vi "OpenDoc Browser.vi"(8 "error in (no error)":errorcluster, 10 "Section":string, 11 "File":path) -> (0 "error out":errorcluster)   [LabVIEW 2019]
doc: "Oppens a PDF document in an external reader, scrolls the document to a given section"
uses:
  <vilib>/registry/registry.llb/Registry RtKey.ctl
  <vilib>/registry/registry.llb/Read Registry Value Simple STR.vi
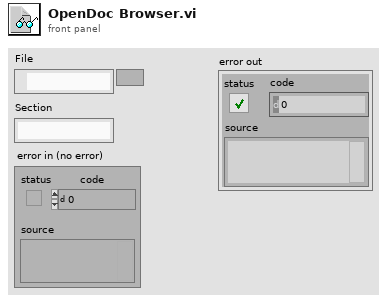
[diagram p1: front panel]
types:
  T1 = typedef "Registry RtKey.ctl" = enum32{"HKEY_CLASSES_ROOT", "HKEY_CURRENT_USER", "HKEY_LOCAL_MACHINE", "HKEY_USERS", "HKEY_PERFORMANCE_DATA", "HKEY_CURRENT_CONFIG", "HKEY_DYN_DATA"}
  T2 = typedef "Registry refnum.ctl" = refnum<k1>
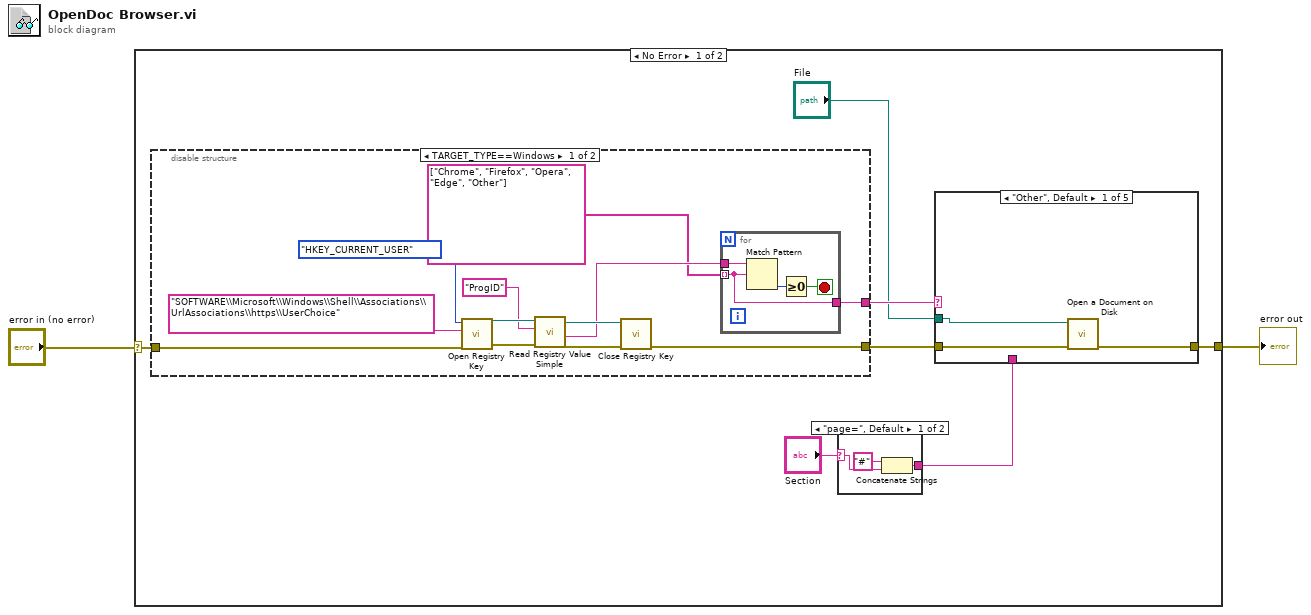
[diagram p0: block diagram]
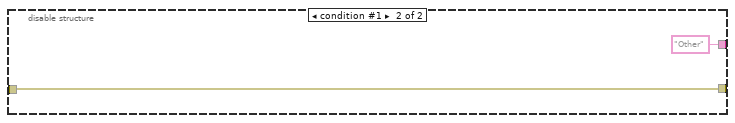
[diagram p2: hidden frame]
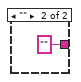
[diagram p3: hidden frame]
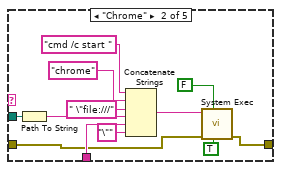
[diagram p4: hidden frame]
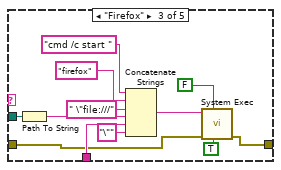
[diagram p5: hidden frame]
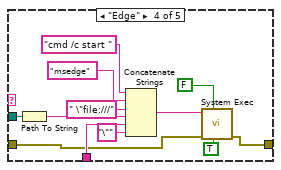
[diagram p6: hidden frame]
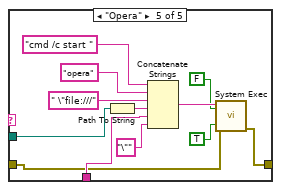
[diagram p7: hidden frame]
diagram:
  n1 = case shown="No Error" "error in (no error)" {
    selector: "error in (no error)" -> [w3 w83]
    tunnel: [w4 w83] -> w2
    frame No Error {
      n2 = disable-structure shown="TARGET_TYPE==Windows" {
        disable-tunnel: [w12 "Other" ("regular expression")] -> w9
        disable-tunnel: [w11 w27] -> w5
        disable-tunnel: w3 -> [w10 w27]
        frame condition #0 (active) {
          n3 = call <vilib>:"Open Registry Key.vi"("error in (no error)"=w10, "subkey"="SOFTWARE\\Microsoft\\Windows\\Shell\\Associations\\UrlAssociations\\https\\UserChoice", "root key (HKEY_LOCAL_MACHINE)"=Registry_RtKey."HKEY_CURRENT_USER") -> ("error out"=w18:errorcluster, "refnum out"=w19:T2)  [unwired: 7 in]
          n4 = call-poly <vilib>:"Read Registry Value Simple.vi"("error in (no error)"=w18, "value"="ProgID", "refnum"=w19) -> ("error out"=w16:errorcluster, "String/Binary data"=w14:string, "refnum out"=w15:T2)  [unwired: 3 in, 1 out]
          n5 = call <vilib>:"Close Registry Key.vi"("error in (no error)"=w16, "refnum"=w15) -> ("error out"=w11:errorcluster)  [unwired: 5 in]
          n6 = for {
            tunnel: w14 -> [w25]
            tunnel: string[] ["Chrome", "Firefox", "Opera", "Edge", "Other"] ("regular expression") -> [w24] mode=indexing
            tunnel: [w24] -> w12
            stop <- w22 stop-if-true
            n7 = Match Pattern(string=w25, regular expression=w24) -> (offset past match=w23:i32)  [unwired: 1 in, 3 out]
            n8 = Greater Or Equal To 0?(x=w23) -> (x >= 0?=w22:bool)
          }
        }
        frame condition #1 {
        }
      }
      n9 = case shown="\"page=\", Default" "Section" {
        selector: "Section" -> [w30 _]
        tunnel: [w28 ""] -> w7
        frame "page=", Default {
          n10 = Concatenate Strings("#" ("string"), w30) -> (w28:string)
        }
        frame "" {
        }
      }
      n11 = case shown="\"Other\", Default" w9 {
        tunnel: w7 -> [_ w44 w56 w68 w80]
        tunnel: "File" -> [w33 w42 w54 w66 w78]
        tunnel: w5 -> [w34 w36 w48 w60 w72]
        tunnel: [w32 w35 w47 w59 w71] -> w4
        frame "Other", Default {
          n12 = call <vilib>:"Open a Document on Disk.vi"("error in (no error)"=w34, "document path"=w33) -> ("error out"=w32:errorcluster)  [unwired: 5 in]
        }
        frame "Chrome" {
          n13 = Path To String(path=w42) -> (string=w45:string)
          n14 = Concatenate Strings("cmd /c start " ("command line"), "chrome" ("string"), " \"file:///" ("string"), w45, w44, "\"" ("string")) -> (w40:string)
          n15 = call <vilib>:"System Exec.vi"("run minimized? (F)"=TRUE, "wait until completion? (T)"=FALSE, "error in (no error)"=w36, "command line"=w40) -> ("error out"=w35:errorcluster)  [unwired: 4 in, 3 out]
        }
        frame "Firefox" {
          n16 = Path To String(path=w54) -> (string=w57:string)
          n17 = Concatenate Strings("cmd /c start " ("command line"), "firefox" ("string"), " \"file:///" ("string"), w57, w56, "\"" ("string")) -> (w52:string)
          n18 = call <vilib>:"System Exec.vi"("run minimized? (F)"=TRUE, "wait until completion? (T)"=FALSE, "error in (no error)"=w48, "command line"=w52) -> ("error out"=w47:errorcluster)  [unwired: 4 in, 3 out]
        }
        frame "Edge" {
          n19 = Path To String(path=w66) -> (string=w69:string)
          n20 = Concatenate Strings("cmd /c start " ("command line"), "msedge" ("string"), " \"file:///" ("string"), w69, w68, "\"" ("string")) -> (w64:string)
          n21 = call <vilib>:"System Exec.vi"("run minimized? (F)"=TRUE, "wait until completion? (T)"=FALSE, "error in (no error)"=w60, "command line"=w64) -> ("error out"=w59:errorcluster)  [unwired: 4 in, 3 out]
        }
        frame "Opera" {
          n22 = Path To String(path=w78) -> (string=w81:string)
          n23 = Concatenate Strings("cmd /c start " ("command line"), "opera" ("string"), " \"file:///" ("string"), w81, w80, "\"" ("string")) -> (w76:string)
          n24 = call <vilib>:"System Exec.vi"("run minimized? (F)"=TRUE, "wait until completion? (T)"=FALSE, "error in (no error)"=w72, "command line"=w76) -> ("error out"=w71:errorcluster)  [unwired: 4 in, 3 out]
        }
      }
    }
    frame Error {
    }
  }
  "error out" <- w2
